vi "MHL_previous file.vi"(0 "Delacor_lib_QMH_Message Queue in":refnum<class "Delacor_lib_QMH_Message Queue.lvclass">, 1 "Data Cluster in":T1, 5 "error in (no error)":errorcluster) -> (14 "Data Cluster out":T1, 19 "error out":errorcluster)   [LabVIEW 2019, in "Main UI.lvlib"]
uses:
  Main UI.lvlib
  <vilib>/Delacor/Delacor QMH/Libraries/Message Queue_class/Delacor_lib_QMH_Message Queue.lvclass
  Module Data--cluster.ctl
  Neo-Laura-LVOOP/Class Library/XYgraph_class/XYgraph.lvclass
  FileReader/FPref_clustered--cluster references.ctl
  Main UI Shared/Boolean--FP cluster.ctl
  FileReader/FPref_cntrls--cluster references.ctl
  Main UI Shared/Indicators--FP cluster.ctl
  <vilib>/Delacor/Delacor QMH/Libraries/Message Queue_class/Delacor_lib_QMH_Message Queue.lvclass/Delacor_lib_QMH_Message Queue.ctl
  <vilib>/Delacor/Delacor QMH/Libraries/Message Queue_class/Delacor_lib_QMH_Enqueue Message (Single).vi
  Main UI Shared/MAIN UI Shared.lvlib
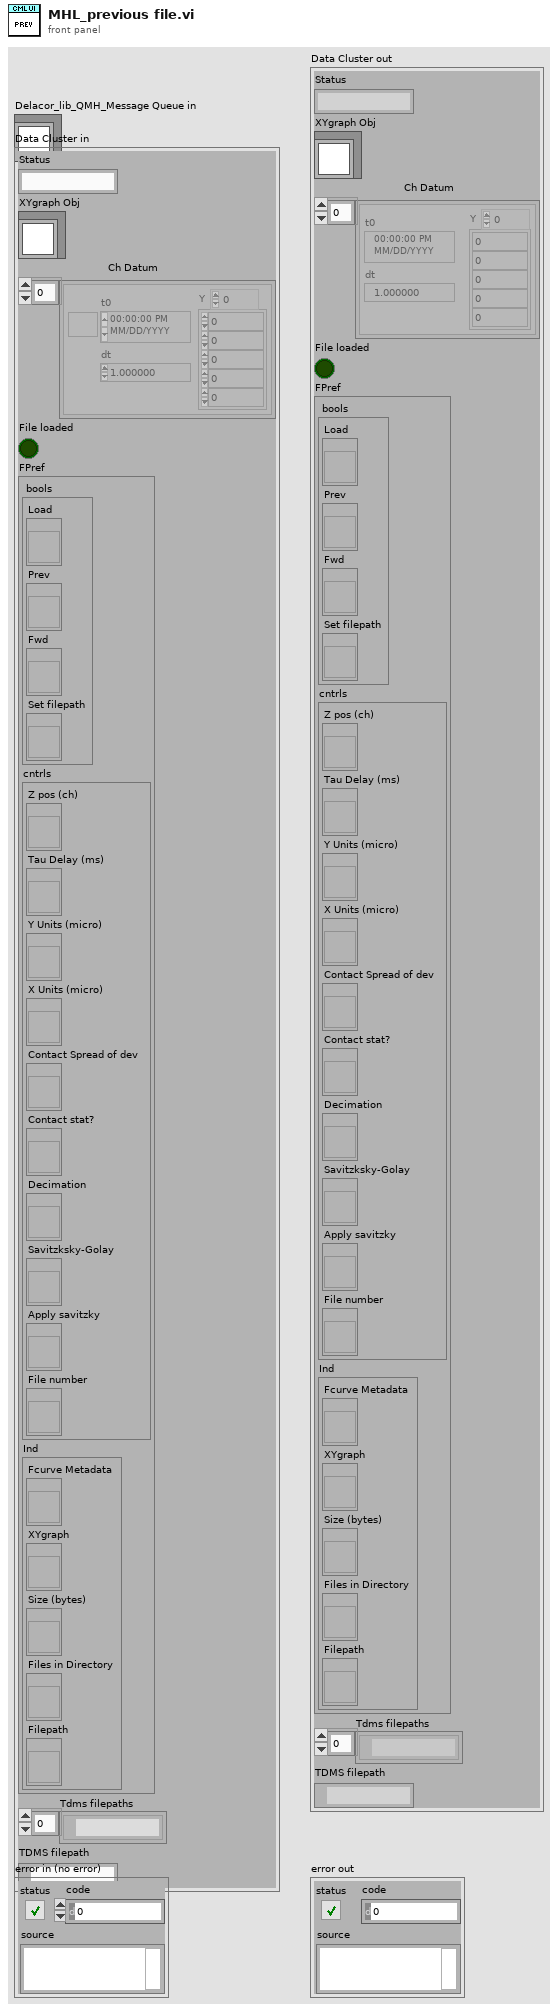
[diagram p1: front panel]
types:
  T1 = typedef "Main UI.lvlib/Module Data--cluster.ctl" = cluster{"Status":string, "XYgraph Obj":refnum<class "XYgraph.lvclass">, "Ch Datum":waveform(dbl)[], "File loaded":bool, "FPref":T2, "Tdms filepaths":path[], "TDMS filepath":path}
  T2 = typedef "FPref_clustered--cluster references.ctl" = cluster{" bools":T3, "cntrls":T4, "Ind":T5}
  T3 = typedef "MAIN UI Shared.lvlib/Boolean--FP cluster.ctl" = cluster{"Load":refnum<vi>, "Prev":refnum<vi>, "Fwd":refnum<vi>, "Set filepath":refnum<vi>}
  T4 = typedef "FPref_cntrls--cluster references.ctl" = cluster{"Z pos (ch)":refnum<vi>, "Tau Delay (ms)":refnum<vi>, "Y Units (micro)":refnum<vi>, "X Units (micro)":refnum<vi>, "Contact Spread of dev":refnum<vi>, "Contact stat?":refnum<vi>, "Decimation":refnum<vi>, "Savitzksky-Golay":refnum<vi>, "Apply savitzky ":refnum<vi>, "File number":refnum<vi>}
  T5 = typedef "Indicators--FP cluster.ctl" = cluster{"Fcurve Metadata":refnum<vi>, "XYgraph":refnum<vi>, "Size (bytes)":refnum<vi>, "Files in Directory":refnum<vi>, "Filepath":refnum<vi>}
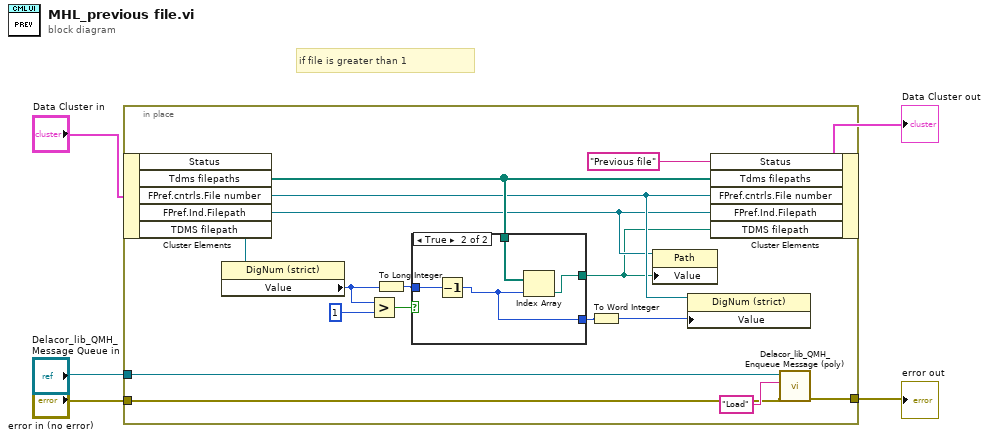
[diagram p0: block diagram]
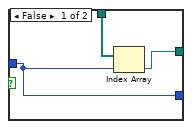
[diagram p2: hidden frame]
diagram:
  # "if file is greater than 1"
  n1 = in-place {
    in-place-border: "error in (no error)" -> [w19]
    in-place-border: [w18] -> w2
    in-place-border: "Delacor_lib_QMH_Message Queue in" -> [w16]
    n2 = in-place-cluster #1("Data Cluster in") -> ("Tdms filepaths"=w15:path[], "FPref.cntrls.File number"=w10:refnum<vi>, "FPref.Ind.Filepath"=w9:refnum<vi>)  [unwired: 2 out]
    n3 = property class="DigNum (strict)"(reference=w10) -> ("Value"=w14:i16)  [unwired: 1 in, 2 out]
    n4 = Greater?(x=w14, y=i16 1) -> (0:w12:bool)
    n5 = To Long Integer(number=w14) -> (32bit integer=w11:i32)
    n6 = case shown="True" w12 {
      tunnel: w15 -> [w23 w27]
      tunnel: w11 -> [w21 w26]
      tunnel: [w21 w25] -> w7
      tunnel: [w22 w24] -> w8
      frame False {
        n7 = Index Array(array=w23, index=w21) -> (element=w22:path)
      }
      frame True {
        n8 = Decrement(x=w26) -> (x-1=w25:i32)
        n9 = Index Array(array=w27, index=w25) -> (element=w24:path)
      }
    }
    n10 = To Word Integer(number=w7) -> (16bit integer=w6:i16)
    n11 = property class="Path"(reference=w9, "Value"=w8) -> ()  [unwired: 1 in, 2 out]
    n12 = property class="DigNum (strict)"(reference=w10, "Value"=w6) -> ()  [unwired: 1 in, 2 out]
    n13 = in-place-cluster #1("Status"="Previous file", "Tdms filepaths"=w15, "FPref.cntrls.File number"=w10, "FPref.Ind.Filepath"=w9, "TDMS filepath"=w8) -> (→"Data Cluster out":T1)
    n14 = call-poly <vilib>:"Delacor_lib_QMH_Enqueue Message (poly).vi"("error in"=w19, "Message"="Load", "Message Queue in"=w16) -> ("error out"=w18:errorcluster)  [unwired: 7 in, 1 out]
  }
  "error out" <- w2
